vi "Close all opened modules.vi"(8 "error in":errorcluster, 11 "Project in":refnum<class "Project.lvclass">) -> (0 "error out":errorcluster, 3 "Project out":refnum<class "Project.lvclass">)   [LabVIEW 2020, in "Panther Dashboard.lvlib"]
uses:
  Panther Dashboard.lvlib
  Class/Library/Library.lvclass
  Class/Project/Project.lvclass
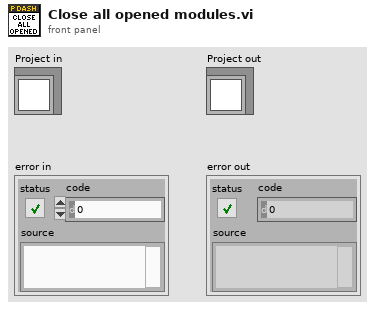
[diagram p1: front panel]
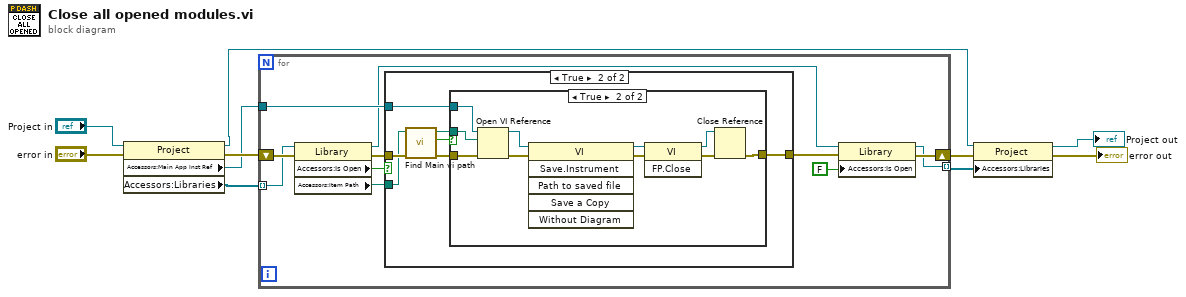
[diagram p0: block diagram]
diagram:
  n1 = property class="Project"(reference="Project in", error in="error in") -> (reference out=w3:refnum<class "Project.lvclass">, error out=w10:errorcluster, "Accessors:Main App Inst Ref"=w4:refnum<vi>, "Accessors:Libraries"=w5:refnum<class "Library.lvclass">[])
  n2 = for {
    tunnel: w5 -> [w17] mode=indexing
    tunnel: w4 -> [w14]
    shift-right: [w18] -> w8
    shift-left: w10 -> [w20]
    tunnel: [w11] -> w2 mode=indexing
    n3 = property class="Library"(reference=w17, error in=w20) -> (reference out=w12:refnum<class "Library.lvclass">, error out=w21:errorcluster, "Accessors:Is Open"=w16:bool, "Accessors:Item Path"=w15:path)
    n4 = case shown="True" w16 {
      tunnel: w15 -> [_ w26]
      tunnel: w14 -> [_ w23]
      tunnel: w21 -> [w22 w28]
      tunnel: [w22 w27] -> w19
      frame False {
      }
      frame True {
        n5 = call "Find Main vi path.vi"("error in"=w28, "Library Path"=w26) -> ("error out"=w29:errorcluster, "Main.vi Found?"=w25:bool, "Main vi Path"=w24:path)  [unwired: 7 in]
        n6 = case shown="True" w25 {
          tunnel: w24 -> [_ w34]
          tunnel: w23 -> [_ w35]
          tunnel: w29 -> [w30 w40]
          tunnel: [w30 w36] -> w27
          frame False {
          }
          frame True {
            n7 = Open VI Reference(application reference (local)=w35, vi path=w34, error in (no error)=w40) -> (vi reference=w33:refnum<vi>, error out=w39:errorcluster)  [unwired: 3 in]
            n8 = invoke class="VI" method="Save.Instrument"(reference=w33, error in=w39) -> (reference out=w32:refnum<vi>, error out=w38:errorcluster)  [unwired: 4 in, 4 out]
            n9 = invoke class="VI" method="FP.Close"(reference=w32, error in=w38) -> (reference out=w31:refnum<vi>, error out=w37:errorcluster)  [unwired: 1 in, 1 out]
            n10 = Close Reference(reference=w31, error in (no error)=w37) -> (error out=w36:errorcluster)
          }
        }
      }
    }
    n11 = property class="Library"(reference=w12, error in=w19, "Accessors:Is Open"=FALSE ("Is Open")) -> (reference out=w11:refnum<class "Library.lvclass">, error out=w18:errorcluster)
  }
  n12 = property class="Project"(reference=w3, error in=w8, "Accessors:Libraries"=w2) -> (reference out=→"Project out":refnum<class "Project.lvclass">, error out=→"error out":errorcluster)
